vi "Set extenstion bytes and type.vi"(7 "Ext size":T1, 8 "error in":errorcluster, 9 "Payload bytes":u8[](array[numeric]), 10 "Payload Ext Type":i8, 11 "MsgPackExt in":refnum<class "MsgPackExt.lvclass">) -> (0 "error out":errorcluster, 3 "MsgPackExt out":refnum<class "MsgPackExt.lvclass">)   [LabVIEW 2020, in "MessagePack.lvlib" / "MsgPackExt.lvclass"]
uses:
  MsgPackExt.lvclass
  MsgPackExt.lvclass/MsgPackExt.ctl
  Typedefs/MsgPack Object Types.ctl
  MessagePack.lvlib
  Requested ext size.ctl
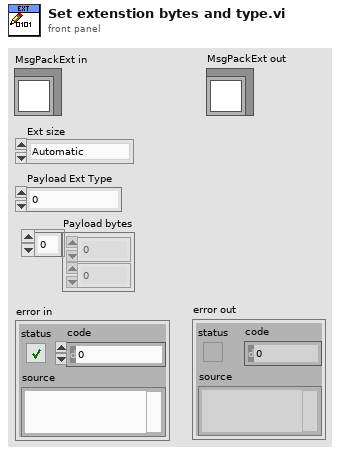
[diagram p1: front panel]
types:
  T1 = typedef "MessagePack.lvlib/MsgPackExt.lvclass/Requested ext size.ctl" = enum16{"Automatic", "Fixed 1-byte", "Fixed 2-bytes", "Fixed 4-bytes", "Fixed 8-bytes", "Fixed 16-bytes", "Up to 8 bytes", "Up to 16 bytes", "Up to 32 bytes"}
  T2 = typedef "MessagePack.lvlib/MsgPack Object Types.ctl" = enum16{"UNSUPPORTED", "POSINT", "NEGINT", "FIXMAP", "FIXARRAY", "FIXSTR", "NIL", "FALSE", "TRUE", "BIN8", "BIN16", "BIN32", "EXT8", "EXT16", "EXT32", "FLOAT32", "FLOAT64", "UINT8", "UINT16", "UINT32", "UINT64", "INT8", "INT16", "INT32", "INT64", "FIXEXT1", "FIXEXT2", "FIXEXT4", "FIXEXT8", "FIXEXT16", "STR8", "STR16", "STR32", "ARRAY16", "ARRAY32", "MAP16", "MAP32"}
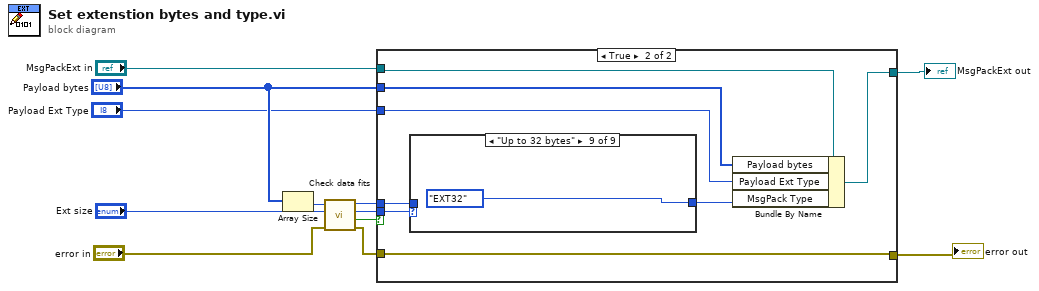
[diagram p0: block diagram]
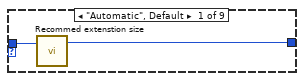
[diagram p3: hidden frame]
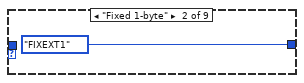
[diagram p4: hidden frame]
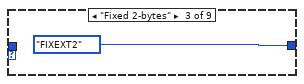
[diagram p5: hidden frame]
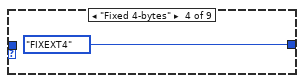
[diagram p6: hidden frame]
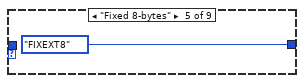
[diagram p7: hidden frame]
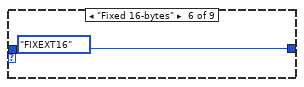
[diagram p8: hidden frame]
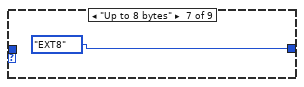
[diagram p9: hidden frame]
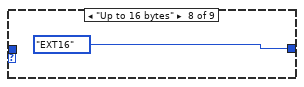
[diagram p10: hidden frame]
diagram:
  n1 = Array Size(array="Payload bytes") -> (size(s)=w10:i32)
  n2 = call "Check data fits.vi"("error in"="error in", "Ext size"="Ext size", "size"=w10) -> ("error out"=w3:errorcluster, "Fits?"=w1:bool, "Ext size"=w7:T1, "size"=w8:u32)  [unwired: 5 in]
  n3 = case shown="True" w1 {
    tunnel: [w13 w22] -> w12
    tunnel: [w14 w18] -> w11
    tunnel: w8 -> [_ w21]
    tunnel: w7 -> [_ w20]
    tunnel: "Payload bytes" -> [_ w19]
    tunnel: "Payload Ext Type" -> [_ w17]
    tunnel: "MsgPackExt in" -> [w13 w15]
    tunnel: w3 -> [w14 w18]
    frame False {
    }
    frame True {
      n4 = case shown="\"Up to 32 bytes\"" w20 {
        tunnel: [w24 MsgPack_Object_Types."FIXEXT1" ("MsgPack Type") MsgPack_Object_Types."FIXEXT2" ("MsgPack Type") MsgPack_Object_Types."FIXEXT4" ("MsgPack Type") MsgPack_Object_Types."FIXEXT8" ("MsgPack Type") MsgPack_Object_Types."FIXEXT16" ("MsgPack Type") MsgPack_Object_Types."EXT8" ("MsgPack Type") MsgPack_Object_Types."EXT16" ("MsgPack Type") MsgPack_Object_Types."EXT32" ("MsgPack Type")] -> w16
        tunnel: w21 -> [w23 _ _ _ _ _ _ _ _]
        frame "Automatic", Default {
          n5 = call "Recommed extenstion size.vi"("size"=w23) -> ("MsgPack Type"=w24:T2)  [unwired: 2 in]
        }
        frame "Fixed 1-byte" {
        }
        frame "Fixed 2-bytes" {
        }
        frame "Fixed 4-bytes" {
        }
        frame "Fixed 8-bytes" {
        }
        frame "Fixed 16-bytes" {
        }
        frame "Up to 8 bytes" {
        }
        frame "Up to 16 bytes" {
        }
        frame "Up to 32 bytes" {
        }
      }
      n6 = Bundle By Name(cluster=w15, "Payload bytes"=w19, "Payload Ext Type"=w17, "MsgPack Type"=w16) -> (w22:refnum<class "MsgPackExt.lvclass">)
    }
  }
  "error out" <- w11
  "MsgPackExt out" <- w12
